vi "DetectCollision.vi"(0 "Goal":dbl[](array[numeric]), 4 "Initial State":dbl[](array[numeric]), 6 "enemy_robots":T1[](array[typedef]), 7 "Robot in":T1, 9 "Is not first robot?":bool, 10 "element being analyzed":dbl[](array[numeric]), 11 "element already in path":dbl[](array[numeric])) -> (3 "Is there colision?":bool)   [LabVIEW 2017]
uses:
  Core/AI Robot.ctl
  Intel/Functions Enum.ctl
  Intel/AttackerStates.ctl
  <vilib>/Analysis/_algsub.llb/Real Vector Norm.vi
  <vilib>/Analysis/baseanly.llb/Real Dot Product.vi
  <vilib>/Analysis/NI_AALBase.lvlib
  <vilib>/Analysis/NI_AALPro.lvlib
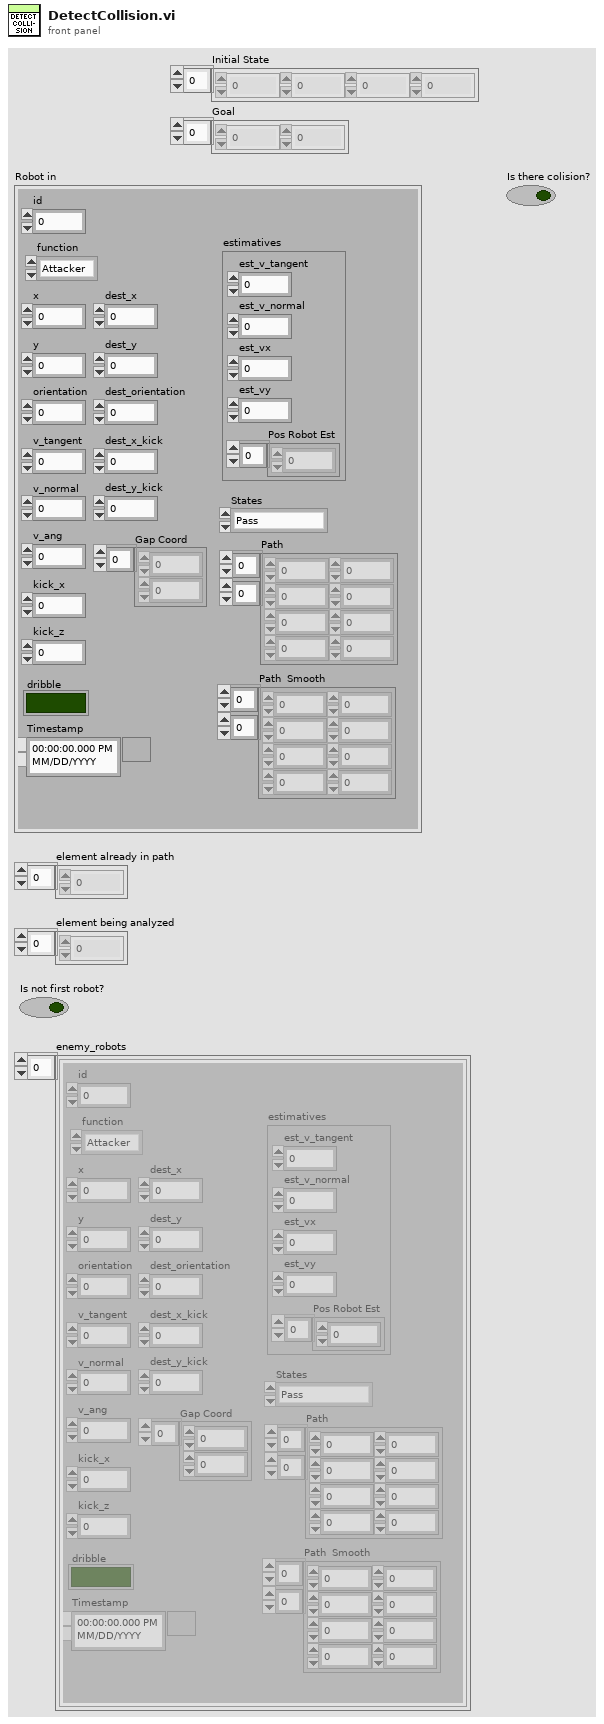
[diagram p1: front panel]
types:
  T1 = typedef "AI Robot.ctl" = cluster{"id":u32, "function":T2, "x":dbl, "y":dbl, "orientation":dbl, "v_tangent":dbl, "v_normal":dbl, "v_ang":dbl, "kick_x":dbl, "kick_z":dbl, "dribble":bool, "Timestamp":timestamp, "dest_x":dbl, "dest_y":dbl, "dest_orientation":dbl, "estimatives":cluster{"est_v_tangent":dbl, "est_v_normal":dbl, "est_vx":dbl, "est_vy":dbl, "Pos Robot Est":dbl[]}, "dest_x_kick":dbl, "dest_y_kick":dbl, "Gap Coord":dbl[], "States":T3, "Path ":dbl[][], "Path  Smooth":dbl[][]}
  T2 = typedef "Functions Enum.ctl" = enum16{"Attacker", "Goalie", "Defender", "Striker", "Goto 0", "Dummy", "Kicker", "ZigZag"}
  T3 = typedef "AttackerStates.ctl" = enum16{"Pass", "GoToTangent", "BallGetting", "GoToKick", ""}
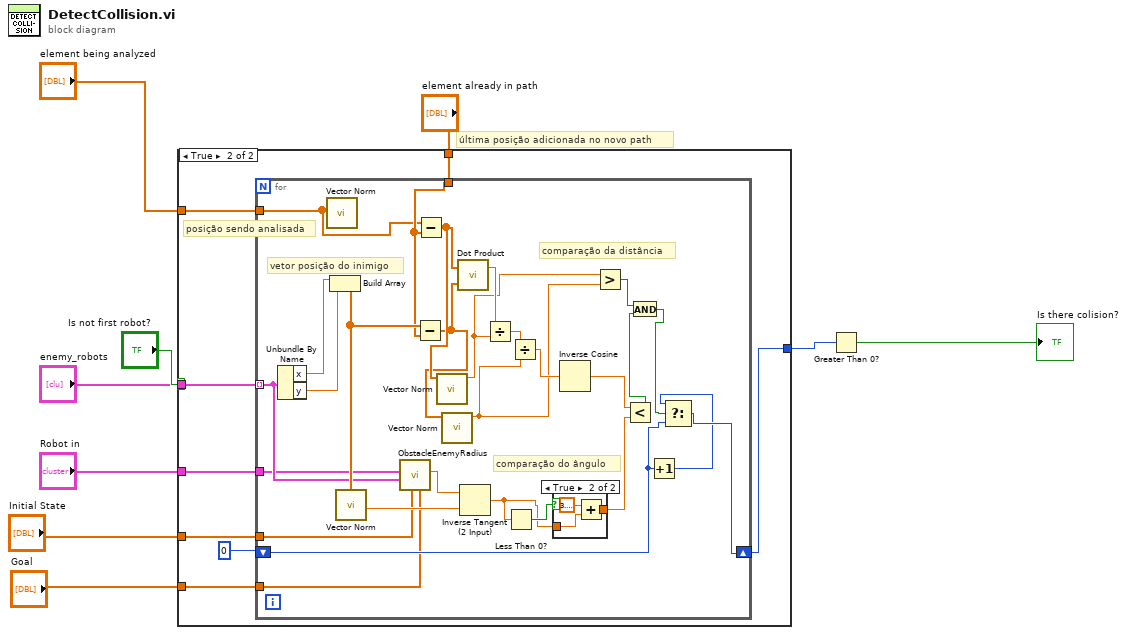
[diagram p0: block diagram]
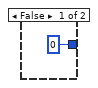
[diagram p2: hidden frame]
diagram:
  # "última posição adicionada no novo path"
  n1 = case shown="True" "Is not first robot?" {
    tunnel: "enemy_robots" -> [_ w18]
    tunnel: "element being analyzed" -> [_ w16]
    tunnel: "element already in path" -> [_ w15]
    tunnel: [0 w14] -> w6
    tunnel: "Robot in" -> [_ w13]
    tunnel: "Initial State" -> [_ w12]
    tunnel: "Goal" -> [_ w11]
    frame False {
    }
    frame True {
      # "posição sendo analisada"
      n2 = for {
        tunnel: w18 -> [w22] mode=indexing
        shift-right: [w34] -> w14
        shift-left: 0 -> [w32]
        tunnel: w16 -> [w41]
        tunnel: w15 -> [w42]
        tunnel: w13 -> [w21]
        tunnel: w12 -> [w20]
        tunnel: w11 -> [w19]
        # "comparação do ângulo"
        # "comparação da distância"
        # "vetor posição do inimigo"
        n3 = Unbundle By Name(w22) -> ("x"=w46:dbl, "y"=w45:dbl)
        n4 = call-poly <vilib>:"Vector Norm.vi"("Input Vector"=w41) -> ()  [unwired: 9 in, 2 out]
        n5 = Build Array(w46, w45) -> (w43:dbl[])
        n6 = call-poly <vilib>:"Vector Norm.vi"("Input Vector"=w43) -> ("norm"=w44:dbl)  [unwired: 9 in, 1 out]
        n7 = call "ObstacleEnemyRadius.vi"("Goal"=w19, "Initial State"=w20, "Robot enemy"=w22, "Robot in"=w21) -> ("obstacle enemy radius"=w23:dbl)  [unwired: 7 in]
        n8 = Subtract(x=w43, y=w42) -> (x-y=w35:dbl[])
        n9 = Subtract(x=w41, y=w42) -> (x-y=w39:dbl[])
        n10 = call-poly <vilib>:"Vector Norm.vi"("Input Vector"=w39) -> ("norm"=w31:dbl)  [unwired: 9 in, 1 out]
        n11 = call-poly <vilib>:"Vector Norm.vi"("Input Vector"=w35) -> ("norm"=w30:dbl)  [unwired: 9 in, 1 out]
        n12 = call-poly <vilib>:"Dot Product.vi"("Y Vector"=w35, "X Vector"=w39) -> ("X * Y"=w40:dbl)  [unwired: 1 out]
        n13 = Inverse Tangent (2 Input)(1:w44, 2:w23) -> (0:w25:dbl)
        n14 = Divide(x=w40, y=w31) -> (x/y=w38:dbl)
        n15 = Less Than 0?(x=w25) -> (x < 0?=w26:bool)
        n16 = Divide(x=w38, y=w30) -> (x/y=w37:dbl)
        n17 = case shown="True" w26 {
          tunnel: w25 -> [w47 w49]
          tunnel: [w47 w48] -> w24
          frame False {
          }
          frame True {
            n18 = Add(x=3.141592653589793, y=w49) -> (x+y=w48:dbl)
          }
        }
        n19 = Inverse Cosine(1:w37) -> (0:w36:dbl)
        n20 = Greater?(x=w31, y=w30) -> (0:w29:bool)
        n21 = Less?(x=w36, y=w24) -> (x < y?=w28:bool)
        n22 = And(x=w29, y=w28) -> (x .and. y?=w27:bool)
        n23 = Increment(x=w32) -> (x+1=w33:i32)
        n24 = Select(t=w33, s=w27, f=w32) -> (s? t:f=w34:i32)
      }
    }
  }
  n25 = Greater Than 0?(x=w6) -> (x > 0?=→"Is there colision?":bool)
